vi "UsrProfiles-Save Load MovCor settings.vi"(6 "Which file? (User profile.ini)":T1=enum."Loaded User profile.ini", 8 "error in (no error)":errorcluster, 11 "Function":T2) -> (0 "error out":errorcluster)   [LabVIEW 2017]
uses:
  Typedefs/Save-Load enum.ctl
  Typedefs/Which path.ctl
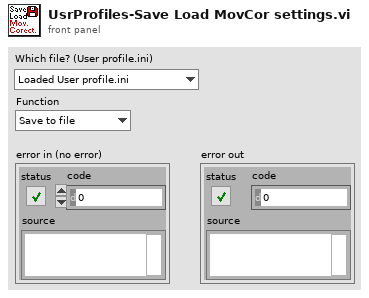
[diagram p1: front panel]
types:
  T1 = typedef "Which path.ctl" = enum16{"Configuration Files", "Calibration Files", "Images", "Setup.ini", "Loaded User profile.ini", "User's-Previous session.ini", "New user profile.ini", "Selected User profile.ini", "User profiles folder", "Power meter scaling.txt", "FOV Cal.ini"}
  T2 = typedef "Save-Load enum.ctl" = enum16{"Save to file", "Load from file", "Compare from file"}
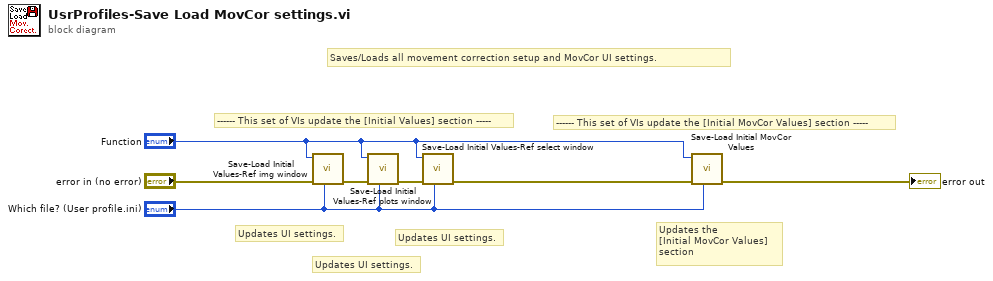
[diagram p0: block diagram]
diagram:
  # "------ This set of VIs update the [Initial MovCor Values] section -----"
  # "Updates UI settings."
  # "Updates UI settings."
  # "------ This set of VIs update the [Initial Values] section -----"
  # "Updates UI settings."
  # "Updates the\n[Initial MovCor Values]\nsection"
  # "Saves/Loads all movement correction setup and MovCor UI settings."
  n1 = call "Save-Load Initial Values-Ref img window.vi"("Which file? (User profile.ini)"="Which file? (User profile.ini)", "error in"="error in (no error)", "Function"="Function") -> ("error out"=w4:errorcluster)  [unwired: 8 in]
  n2 = call "Save-Load Initial Values-Ref plots window.vi"("Which file? (User profile.ini)"="Which file? (User profile.ini)", "error in"=w4, "Function"="Function") -> ("error out"=w3:errorcluster)  [unwired: 8 in]
  n3 = call "Save-Load Initial Values-Ref select window.vi"("Which file? (User profile.ini)"="Which file? (User profile.ini)", "error in"=w3, "Function"="Function") -> ("error out"=w2:errorcluster)  [unwired: 8 in]
  n4 = call "Save-Load Initial MovCor Values.vi"("Which file? (User profile.ini)"="Which file? (User profile.ini)", "error in"=w2, "Function"="Function") -> ("error out"=→"error out":errorcluster)  [unwired: 8 in]
